vi "Main_15B.vi"() -> ()   [LabVIEW 2024]
uses:
  Utility/Universal Utility/TypeDefs_Utility/Cluster_Row-Column.ctl
  Utility/Universal Utility/TypeDefs_Utility/ENUM_4 Directions U-D-L-R.ctl
  Problem-06_Guard Gallivant/ENUM_Direction.ctl
  b5234449-2328-4583-8824-3fa0b55a92a1.vi
  51507f66-8fb0-4352-a9b4-7069ff2e9da3.vi
  afbcc12a-728a-4e4e-a13e-cfea6d256629.vi
  <vilib>/Utility/error.llb/Trim Whitespace.vi
  <vilib>/Utility/error.llb/Trim Whitespace One-Sided.vi
panel:
  out "Direction":T1
  out "Grid Start":string[][](array[string])
  out "Array 2":T1[](array[typedef])
  out "Position":T2
  out "Grid End":string[][](array[string])
  in  "Example 1":string="#######\n#...#.#\n#.....#\n#..OO@#\n#..O..#\n#.....#\n#######\n\n<vv<<^^<<^^"
  in  "Use Puzzle":bool
  out "Answer 1482350":u32
  in  "Puzzle":string="##################################################\n#.......#....O....O......O..O#.OOOO....#.OO......#\n#..O.O..#O..#O..#O.OO......O....O..O....#O.......#\n#...O......O...O...O.......#O#.O.#OO.O........O.O#\n#..O..#O..#.O....OO..OO.....#.OO.....#.O#OOOOO.O.#\n#........O#.....O..OO......#.O..O#...O.O..O......#\n##O..O.O...#O.#...#O...#O..##......#............O#\n#.OO#O.O..O...O#..OO...#..###O....OO.#.O.##....#.#\n#.O...........O.....O..O.OO.O.O...O..OO....OO....#\n#OO..........O...O........O..##O.OOO.O..O..O..#.O#\n#.#O.....O.OO....#O..O...O.....O...........OO..#O#\n##.....O.......O.O.O....O.O...#O.O..O##....OO#...#\n#.OO......O.......O..#...O......#.OOOO.OOO...#O..#\n#.........O.O....OO..##.....OO...#....O.OO..OO...#\n#O....O..O..#...OOO...OOO#..OO......OO..O....OO.O#\n#....O.........O....#.#.O..OO......O.O..#O.O#OO..#\n#...O.OOO.O.O..O.........O.OO....OO.O.....OO..OOO#\n#..O.........#...OO.O#.O....OOO......O..........O#\n#........O.O.O.O..OOOOO.#.O.OO#OO.....#...O.O.#O.#\n#OO...O.#O.OOO....O....O.#.O.OOO.O..O......OOOO.O#\n#...#OO.O..O...O.OOO.....O.O.OO.#..O#...O..OO....#\n#O.OOOO.O........#O.##......#....#...OO..O.O.OO..#\n#.OOO.O.O#OO...O.O...O.........O........O..O#OOO.#\n#.#..O........#......O......O.....O....O.#..O....#\n#...#.....O.O.OOO.OO.O.O@O.O.O.O..#O....#.#.OO..O#\n#O.......#O...#O....O.#.....OO.#O.O..O.O......O..#\n#......O...OO.OO..O#....OOO.#.#....O.O....OO....O#\n#...O.O.#..OO#.O.OO...O.#.#..#O..#...##..O.......#\n##O...O..OO.O..O.OOO..O.........O#O...#..#.O..O#O#\n#O.O....#OO..OOO.#O..#O..O.#...#.#..O....O.O....##\n#.O.OOO.O....O...#O.O...OOO..O.....O.O..O.O..O..O#\n#......O...O..OO.O........O..........O....#....OO#\n#.O..OO.O.OOO..OO...........O........O.O....OO.O##\n#.O.OO#....#.........#..O...OO...OO..OO..........#\n#...OO...OO..OO.O...O.....#...O.#.....OO.O.O.O#O.#\n#OO......#...OO......O..O.O...O...#.....O......OO#\n#O...O.....O...O.O.O....O##OO.O..#..O....O#OO...O#\n#.O.O#OO..##.#O...O#O..O.O#..O...OO...OOO.......##\n#...O.#.O.#......OO.......O.OO..#.OOOOO...OO..O.##\n#............O..O.....#O.##.O.O.#....O#.......O.O#\n#.O..##..O....#O.O..#....O...OOO#.#...#..O...O...#\n#.O.OOOO..#.........O.O#....O....OO.OO.....##OOO.#\n#..O#...OO..O...O#...#..OO.OO...#....O........O.O#\n#.O.O..O....O...O.O.OO#...OO..O.OO.O.O..O...O....#\n#.O#..OO...#.OO...........OO.....OO#O.#..O.O...#.#\n#..................O.......O...OO..O..O.O.O.O##..#\n#.##.#..OO.#..........O#...O.O.O...##..O......O.O#\n#OO.O........####.......O.......O......O...##....#\n#.O........O..O..#...O.OO...#....#.#.....OO...O.##\n##################################################\n\n<><v>^vv<^<v<>^>^^<^^>>^>><vv^>^>^<v<>>^^>>v^>^<v><v><v>>^<^<<^^>^>^<<v^<<^^v><<><v>v^>^^<v<<<>v<>^>^^^><v<><v^<><vv^v>^>^>><^<vv<^>^<^<<<<<^<^vv><v>^v^^><<>>v<v>vvv^<>v<>v><<<v^<^<^vv<^v<>v<<<<<>v<^<<<^<^v^<^>^>>vv>>^^<>^^<^v<^v<<vv<vvv^<^^<>v^^><^^^v^>^>^^<<<^<v<^<><v^<^v^<>>v><^^v^vv><vv>^v>>^vv>v><v<>>>^>>^v>v^^<vv^<v>vv<^<>^>>^v^v><^v^>>^>^<<<<<><v<v<vvv><><^^v^^^<>v<>vv>v^>>>^<>>^^^><v<^<>v<^>^<vvv^>^>vvv>>v<>v<>v<><><<^vv>^<^<<>^^<v<^^>v^v<v<>>^^><>^>>>^v^<>^^^<>><v><>v><>v>^<>vvv>>><><v<><>v^vv^>v^^>>v<^<^<v^>>>^^>>v<<<v^vvvv>^^v>^v<^>^vv^v^v<^^>v>^vv<<v^^^v^<v<^v^<v><v>^^v<^^><^^<^vvv<v<<><>v^<>><<<^vv<^^<<>^^<^<^>^<><v><^>v>><><v^vv<<>>^^>vvv^><<^v<<^>^<^<<><^<>^<>vv>><v>^^<v<v>v^v^^<<>^>>^^v>>v>^^>^<><^>v<vvv>^>v<><vv<><^v>>^<^^<<<<<>^vv<<<v>^<><^<v>v^<v<v<v^<v^<>^v<vv^vv>v^^>v^>^^<v^<<v>^^v>v><<<<<^vv><v>>v><^^^v<^^vvv^^>^^^>vv<>v^<>><><<><^>^^^v^<v>>>v<>vv>vvvv^>>v<<<^vv>>>^v^v><<^vvv^<<>v<><^v><>^v>>v>^^<<>v^vvv><^^<>>^<<<<>>^>>v^^<>>>>vv>v<v^>^<^v>v>>^^>v^^v<^vv><^<^^<vv\n<<^<><v<^vvv<<vv<vv<><v^v><>><<v^<>^>>^>>^^^<^^v<vvv^v>v<>^>><^v>^^vvv^<>>>v>>vvv><^^v>vvv<vv<><v>>vv^^<>^^<^>v^<v>vv^<><v<^<>^vv>^^><>^>^v^<vvv><>^>><^<^>v>v>><v<<vv^^^>^v^vvv>>vv^^<^^<>>v<<vvv^<^<^>>v>>v<<v^<^v><v^><^>v^<v<vvvvv>>>^^v><<^^>v><<<^^<<<^><^<<^v<>^<>v<<<v>v<v<<<^v^^^<v<^^^<^<vv<>>^<^<>v^>>v^v><^vvv>^>>v><<^<<v>v>v>^v<v^<v^^v>^>>^<v^v<>^v><<>>>>>^>^<v<v>>^^v<><><<v>vv><^<>><v>>>v^v<>^><v^v^><<v<^^<vvv<v>^>vvv<>^>>v>^v<^^^v>v>v<>>^<><^<^<<v^<^>vv^v^>v^^^^^v^v><>v<><<<v^vv^>v<v<><>>^^<^<v<>^><>v^^>^^><>v>v^^>v<>>^>^^<v<^^^<<^^>^^>vv<^<^><>^^^v^^^>>^>>v<<^v^^v^<^^^v<^^>>^>^<v<>>^^>><vvv>v<v<>^<vv<v^v>^<v>v>v<>v<v<<<><<<^>>>^>^v>vv>>v^vv^<vv>><<>>v^>^^>>^v>^^v^v^<^<v><><v>v><^^^>^><v>vv<><<^^^<v<^^vv<><v<v>vv^^><><^v^<^v>v<<v>>v<vvv<<^<<v<vvv>>vv<<^<vv><>>v><vv<<>v<vv^><><^v<^<><<>>v<>v^v^<v<><v>^>v>v^vv>v<<v^>>><<<v<^v<v^^v^^>v^v>vvv>v<^v<^<<^>v>><<<v<>>vv>v><vvvvv>vv>v^<^^^<v<v^v<<v^v<^^>>v<vvv<>v>>^<v>^<v^<>^^>>^>vv^<>v^v^<vv^<>>v^^^v^^^^>^v><v<>^>v<v><>>><><^v><^^v<>v^v^>\nvv^^>v^^v<v<vvv<v<<v^>vv<>>>^v^>v>^><>v^><><v^^<^>v><vv>>><v<>v<<<^v<<>^^<vvvv^^>v>v<^>v^^<<vv^v>v^><><><<vvv>v>vv^<<<vv^<v<^>v^<^>vv<>>>vv>^^^^>vv>v^^v<>^^^>v><>>v<>v>>v<^<<>^>><^v<<^<^>><>vv>^><>^^^^^^>^<^<v<<^<<v<v^v>^vvv^<>^v^>><<<^^>^^<v>v^v<^>>><^^<v^<vv><<vvv<<^>v^^>v>v<v^v>v<^v>>v^>^<<v><v>^>^<v<><^>><>>^><^<<^v><^<<>v>><>v<<v<><^v>><^<vv>>v^<><>>^^<<v>>>v^>^v>v>^<v<>><v>^<v<v^^^>^>^vv^<vv<<<>><>><^<v<<<v>>v>^>^>v<><><^v<>><>vvv>^><<^^^<vv<vv><>vv>v^>vv>v><><<^vv>^vvvv<<<<v<v^<>>v>v><v^><v<<v>>^v^^v>^v<<v^^>v>><v<<v<^v<v^^<<<v^^<<v^>^^^^^^<><^>v^><><v^<^^<>>v^<v^v^^^<v^>^^v>v<>^><v>^^><^>^>v>>^<>vv<v<^^v<^^>v^^<>^<^>>>^<^v<vvvv>^<v^>v<<^^^<v<>^v<<<>>^<<^vv>>vvv>v<<>><>^^><vv><<<^v>>><<<vv<v><<v>^v^vv<v>^>>v<<v>v>>><v>><^^v^v^v<<>^>v^>><v^>>v><<vvv^<^vv^v>>^^>v^v<<<>^>v^^v<<vv>v^>v<<^^<<>>v<<v<v^>>^><>^vv^><^>v<<v><<<v<^vvv^v^^v^>><v>vv<>^>v^<<v><><v<^v>v>vv^^v^^<<>>^<v><>v^>>>v<^<vvv<<v<>v>v<v>vvvv>^v>v>^^>v>^><v<^>v><<>><v^vvv<^^v>v^^^^>^<v<>>^>v^<^<>^^>>><v^v>>^><^v^vv>^<v>v<\nv<^^vv><>><<^v^<^v^>^^<^>vv<<^vvvvvv^<><<vv>^<^v>>>><^v<<^<>><>><>>>><<^>>v>>^>^^>^><^<<v^v>v^v>^<^v^<>vv^v>><>vv>><>^<<v><v^v>v>>^^^<<^v><v<v^^>>^vv^>^^>^^v^<<<^>^>^><>v<<<v^>^^^>v<>^<v^v<>>><<<v<>^>v<^^<>^^v<^v>>^>><v<v>>^><^v<^<><>v>v>>>^<<><^^^<<<vvv<^>>^><^><v^<v<v><^v^v<<<><v<vv><<^v<v<<v^^<^<^^^>v^^>v><>^v^><^>>>v>><^v^v>v^<<>v^v<<^<<vv^^<v^^v<>^>^>^<>v>^v<>v>>v>vv^vv>^><><v<^<><<<>>><<>^>^<v<>>>^^<>>^>v^><^vv><^<^>>v>vv<^<v<><^v<^>>><^v<^><v><v^v^<<^><^<><^^<^v^^v>vv^^<v<<>^>>^^v^^<vv<<^vv<vv^<>vv>^>^<v^><><<><<><^v>^^v^><<<v<^<vvv>^><<>>><<v><>vv^^>>^^><<v><^<v>vv^^<^<^^^>^<v<>^v^>v^^v^<>v^<v^v<v><^>v^^><<<>^^^<<v^v<<<<>>v<v^^v^vv^vv^v>v>>^>>^vv^v^<<^vv^<v^v^<>^<^<v>v^<<v<<>^^>><v^>v^^>v^>>>v><<>><v^^^<><><v<<v<<^v>v^>><v<>^vv>^><v<^v>^<>v<<><>>v^v^>^>v>><^<^^><v><^>vv>v<vv^><^^v>^^>v^v<>v<v^^^<<><v>^^vv>v<^>vv^^v^v>>^vv^<><^<^<<<v<>><>>^>^^^^><^v<<<>v^<^^vv><^v>v^vvv><>v>^<<^^^v^^<>>v<^^v<^^^>>^vv<v^^<vvv<^<<^>v^<>^^^<^v^^<v>^><^>^^^v^^>^<>>^v^>vv<v>^<vv^^><^v^^^>v<^v<<>v<^<v\n<^><vv^v^>>^<>>>v><^vv<v^<^vv<<>v^>v<v^^^^>vv^><<v>^^^v<v^<<v<v><^^v>^<v<<^>^^^>v>v<^^>v^v><<vvv^^^>vv^v>^<vvv<vv><<>>>v>v<vv<><<><^v>vv><<^^^vv<><^<<^>^><<>^<v>^>^v<<>>v^<^vvv<v^>>v<<^>^>v<<<^v<><><^^<>^<^<v><<vv<>>^<v^^><^^v<<><vv><^>^^>v^vv^^<>^vv>v^>v>^v>v>^>^>^>><>v<^v>><^<>^v<>vv<^v<^v^<>^<>^<^^v><v^<vv>v<^>>v>>v^v^<^vvv>><v<vvv><<^^<^v<^<vvvvvv<v^^^>^^vv^^v>>>>>^^>v^>^><^><>>^<>v^>v<<<^v><v<v^^vv^<^^v>^v^<vvvv^^<^<^<<<v^v^^<v<<v><^<v><vv<^^>v<vv<^<^v<^>^^^vv^<>^<v>^v^<><>><v>v^<<><^^^>>vv<v^^<v>>^<<>v<vv>^<<v<^<<vv^^<v<vvv>^vv<v^><vv<><v>>^^>v>^<>>^^<v<v<v^<vv>><<^><v<v^<<vv^^^<v><<^<v<<<v>^<vv^><<<^^v<^>vv<>>^>^v^<v>^^v>>v^>>v>vv><<v<<v>v^vv^>vvv^^v<>^>^v><vv>^><v>v^>^v^^><>v<^<v>^<<^vv>^v<<><vv>v^>vv<>>^>>>><<^v<v>^<><v<<<<>>^v>v><^v^^>^<<<v<v^^v^<>v><^>^>^^^v><<<^>v><^><<^vvv<vv^v>v^><<><^>^<<vv^>v><>v>v<>v<vv<>v<<^v>^>^v>^^v<>v>v<<v^v>>>vv>>v>>><^^^v^>>vvv^^vv><^v^<vv^><<^v<vvv<^^v<<vv<<v<><vvv<><<>v<v>^><<>><v<v<>^<v<>vv<<><<v^>^^^^^><<><^v^v<^>v<^^^><<<^<^v><^v<>^>>v^v^<^^\n>vvv^<<>vv>vv<^^vvv>vvvv^<^>v^<vv^^v>^v<<^<<v<<vv>^v^v<<><v<><<>>><><v><<>v<<>>v<<<^>><v<v<>>>>vv>>>>^v<>^><v>>^><v<>^v^v<>^v<^v>^v^^v^^v<><^v<<>^<>><v><^<^<<<><^v^vv<<<<>>>^vv<<><<v^^vv<>vv^>v<^v^>vv<>vv<<v^<>^<<<>^><v<vv><>^v>vv^><<^^<v<<v><>^>>v><>^>vv^^>>^^<^>^^<^vv^^<>><v<<^><<v^^^<v^v<<>>>>^v^<v^>>^><<v^<v^^>>v<<<v>>>^<v^^>v^v<>^>>>>>^^^>v>v>>vv<v^^>>^v>v^^vv<<vvv<<>^^v<<>>>^<><<<>v<>>^v^><<>^>v<>^^^>v>vv<vv>^<^^v<^^>v<^^^^<<<v>><<vv<v>v^>>><v^v>v^^^v<<<v^><>><^<^<^>><>^^v>v>v>>v<>>>v^^><^v<^>><v><v^<^<^>^^^>>>v^<>^>^v^v<vvv<^^^<>><<v<<>><^v>v^v<>>vvv<vv<<><v<>^<<^vv<^vv><>v<^v><^<>>>^<v<vvv<^vv<^vv><^v^><<<v^^<<^v^v>^>v^^^^v<>^^^<<><<vv<<^>vvvv^vv>^<vv<^^<^>^<^^^>v>v^<<>^>^<<v><>^v^^^><<><>v><<<><>v^>v>^<<<>v^>^<<^vv>>>^vvv<>>vv<vvv^<v<>>>v^vvv^v>^>>v<v^>><v^<^<^<^v<vv>v>^><><><^v>>v<^^^v>^vvv^^>>^<^<^^><<>^^<v<<^>^>^>v><>v<<v><<>><^v<>v>^<>^v^>v>^<>^>^>v^<v^><<>><<>v<^v>^<<<<<<v><<>><>><>><^v^^^vv<v^v<vv>v>vv<v^^^v^><v^^v<>v><<>v>>><<v><^<><>^v<v<><<<><>>^<v^<v<v<v^v<v<><v^<>vv\n<<<v^>v>>^>v>v<v<>^^><<^^><^^vvv>>>^>^><<^^<v<><v<<>^^^^vv<^<v^><<v>>><<<<<<<vv<<><v<<<>v<v<<^vv^<v>^^^^^^><^vvv<>v^>^^vv<vv><^>><v<>><>^<<vv^^<>^>^><v><v>v<^v<v<^^^^><^<^^><^v^^<vv^<><<^>^v<v^^v^^<>><<v<^^^<>vv<^^vv^><v><<v^v>>vv^><v<^^^v<<v<<<>vv>>><v<vv>^<^<v<v<>^>v><^>v>v<^<>v^^>>^^<>^<^<v>><<^<<^^^v<v<^<^<<v<v>>^<>><^v^v^<>vv>><v^^><v>><^<^>>^^<<v^<<<>v<^<v^v<v><<^v<vv<v<<>^v^v<<><v^><>><^v^vv^>>v^^v^^^<v><<<v>>^v^><^<v<<>>>^v>^^v<><vv<^^<>^^<<v<<v<<v^^^<^v^<<>vv><<<vv^^<^^vv<^v>^<v>^^^vv^<>v<<>^vv<<vv^^<>v<><^^<vv<<v^<<^<^vv>><^>><>><v^<<v><>^<<^vvv^>v^^>v>v^^^^^^^^v^^^v^<^^^v^^vv^>>v>v^^<v><><<^>v>><^>^v^><^^v>v^vv<v^>^>^<<^^^vvvv<<>><>v<>vv<vvv<<v^^v^^vv><<>^<^>^^^^^vv>^><^^^<<><>^^v^>^^>>v^^^<^<><>^<<>>v^<v<^v<>>>^<vv>^v^>^<<>^v<<v><^v^>><>^<><<v<>><v<>^>^vvv^^>v^>>v>>^>vvvvvv>>v>^vvvv>>^^^<<v>^^^<vvv<<v<v^v^^v<><<<v^v<><<vv<<<<vvv^^^<^>v^v^v^^>^v>^<>^v>>><^vv>vv<^^^vv<>^<><><>vv^v>v>v>>>^v^<^<>^<v<v<v><^<<>^^<^<>^v>>^v^>v^>v^>v<v^>^<>v^<^<^<vvv<v<vv^v<<>>^<^v<^^^<<<^>^^>^<<v>\n^v<v^<^^>>^v><v<><^<><><>v^<>^><>v<<vvv<><>v<><<^^vv>>^^^><^^<>^>><<^^>v><v><^>^>^>><>v^<><><^^^v<^<v^<>v>vv>v>^<><<><^^<^^v<><^<<v^<<^>^^>>>^>>^^^^<^v><><<<^^<^v>v^<^v^><v>^^^><^>^vvv>^v<>v<v><<<^v>^<v<<>^^^<^>^^^<^<v<<>>>>v^>^v^>v^v<v<<^<^^<v^^>v<><^<><^>v^v><<v<v>^vv<^vv><v<v<^><>^v^<<^>vv<^^v<^vv<>>v>>^<>^>>^>>>>^v^<>><v^>vv^^>^v^>^<<<v>^><<>>>><<>^v<<>>>>>^>^^^>>><^>>v^vv^^v><vv>^v^vv^vvv^>^>v>v^vv>^v^^<vvv>vv>><<<<^<<<><>v^v^^^<>^v^<>><<^^^<>vv<<<v>v<<<^>><>^<><v<v>v<v<vv^vv<v^vv^^<<<<vv<>vv^vv<v<<v<v><><>^^><^>^<><^v^>>^<^>>>vv^><<><<^>><v<<v^v<>^v^^v^<><v>^v^^vvv<<v^v<<^^^^^<vvv<><^<>^v<<>><v^v^>>>v^^<^>v<><vv><<<<^<v<v<<<^>v<<<v^v<<^v>^^><<<v>vv<<>v<>v^v<^<>^>>><^v><>^^v><<>vv^v<^v><vvv<<vv<><^>>>v<v><<^^<v>^vv^^>^v<<^<>v^v<v><<>^vv><<<vv^v<>^<v^v<^v>^<<<>^>^vv^><>v^<>v<>>>^vv<vv^<^v^<v><>>v><vv<v>><^v^^^^>>v^>^>v^^<<^^v>vvvvv<>^vv^<^<>^<>v>>vv>v>v<>^><>v^^^vv^>v^<>^vvv<>>>v<<vv<<v>>v>><<^vvv^>v^<<v<v<<>^<><^v<<^>>>v^<^>v<<<<v>^^^^^v><>v>vv<>>^<v^^^v<>v<<>v^<>>v><^^^v^^^>^^>v>\n<>^^<<vvvvv^>vv>>>^<>^v^vv<v^<^v>^^><^>><<^^vv>v<v><v^<^<^>><><<<>v^v>vv<v^v^v>><><v>>^<v^<><v<^^^v<v<<v<<^>^v<^^>^^^vv^><>>^<<<<v<^^<v^<<^^<v>>v^^vvvv^vv>v>>vv<^^>v^vv<>v<v<v<^<v>v^>v^>>^<v><<<<<^^<>>^v^<<v^><v><>vv<v>^^<^<><v<^v<^^vv^<><v>^<<^<>^^^^^>^vv>v>^>>vv>v<>v^^<><^^>^>><>^^v>v><v<^<<<^v<>^>^v^^v>v>>^>^vv><^>^>^<><^^v><v<^>v>vv^v>^v^>^>^v<v>>v>>v^<<v^>v^>v^>>v<^<<<><>^vv<>>v<^^^>v><<<><<<vvv<v<>v<^vv^v<v><^^vvv>^^vv^<>>v>^vv^^<^<>><<>v^v^^^^^<v>v^^<<^^<^v>>>^>^^^^v>^^v><^v^>^v>^^^<>^<<^v^v>v><^^v>^vvv<<>>^v^^>^>^v<v^>>>^v><v<>vv^v>v>v^v<^v>vv>>^>v^<^^^^>^<^>v^^>>^<>^^><v>vv<^>^^<^><<>>^>^v>>v>^<^v<<vvvv^vv<>>v<><^v^v>^v^^v^v<v><<^^v><^>^>^v<vv^^^^<^^v^v<v>^><<<v><<<>^v^>v>vv<^<><^^<>^<>>vv<v<<>^><^^^^v>v<>>v<<>vv^>^vv><<vvv><>v><^v^><vvv>vv<v^<>>^v^^<<<<>>><v<>>^^><^><v<^^<<<<^^^>vv^>^v<<v<vvvv<>^^v>^>v^^><<^<^v><v>^^^>v^<>>^>vv>><^^><^^^>^>><^<>>>>vv><><^<>>v<>v>^v^>^>^><v^^>v>>>^v^vv>v>><>v^^^>><v><>v<>v^^^vv<<vv<vv><><<^<<<>vv<vv>v>^^<v>>v^>>v><<v>^^<><>^>v^<>^vvv>^<^v<<vv<\nv><^^>v>v>^<^<^<<v^<<v><^^<<<^^>><<<^>^^vv<^>vvv<>^^^<<>^vv^v>^^v>^v^^v^<>^vvvv^>vvv>^^<<v>v>^>vvv>><<<v>>v^><>>^<<v^<^^v>><<^^^^><v^<<^^>^^v>^vv^>vvv>v^v^vv^>>^<^<>>v<v^v><<^^^><^^vv^v>v>^>v<v>^><>^<>^>^>vvv>>^<^>^vv>^^<>^^>^><^>^<v<>>^vvv<vv^v>>><<<v^>^v^><^v^<v>vv<<<><<<vv^^vv>>v<v<>v<><^^vv<>>>^v^^<^<<>^<<^<vv^<v>>>v^<>^>>vv>>>^^v^v<vv<^v>v<<^v<^<v^v>v<v>^^><>v^v><<<<v<>>>v^vv<^>>^><v>^v>^<vv<<^>^>v^^<^^^^vv>><v^^v^>^>><^v<^v<>v^>v<<^<v<vv<<^<>vv<>^<v<>^^vv<^^^^<^>^^v>v>v>v<vv>v>v>vv^^<^^<vvvv>v^<^>vv>>>^^^>>>><^^<^<v>v^^v>>>>>v>^>>vv<v^>vv<<<><>v>vv>^><<>>v^<vv<v^v>^v^>>^v^<>^v<^v^<v<^v><^^>v<v<>>><>><^>>^v<>>><><<v>^>^<v><^<^<<v^>v>vv>>vvvv<^>^><>v^<>^><<v^^^^^v>^>v<v^v<>>>^^vv>v>><^^<>><<v>vv<<<>><^v><v>^^<vvv^^^^^<^v>^<<v>>^^vv><<<v<>v^<<><v<>><^<>v<<^v><vv>>^^^v>v><^^<v^><^<v>vv<v^^^^^>><>^^<<>^>>v^^>v^<><>^v<^v>>v^vv<>v<<^<v^v>>^>><v<^^vv<^^<^<v<><^vvvv^>v^<<<><<v>^^^><^><v>^<<^^vv^vv>v>v<^>>>>^v<^v>^v<<^>>>^<<^<v^^v<^<v^<v>^^^vv>^<>^<^<^><vv>>>^<>^^<<<<<v^^>>>vv<^^>>>v^<vv<^\n>>^>^^>vvv<<^^vv^<^>v>^<^<^<^>v^<v>>v>>v>^^>^<<>>vv>>^>>>>>v^<v>><v<>^<vv<>>><v<^^^v<v^<v^>^>>>v>^v^v<^v<>^^v^^^>>>^>v<^>^<<><v<<<<v>v>^<^^^<<>^<v^>>^<<<^>>^>^^>^v^^><vv^<v<v^v^<^>^<v^vv>^><^^^><^v<<>v<^<^<v>^^>v>^v><>^<>v^v^<^<v><>vv<>vvvv<<<^v>v>v^^<<vv<<<<v>>v^^^v>>v><^^^><v<<^v^v>^<<>>><^^v>>^v>><><><<vvv<^^>^vv<^^v<>^vvv><<^^<v>>>^>vvvv^^vv<^v<v<><<vv><><>>>><><v>v^><^vvv>v<<>^^^v>><vv<v<^<v^^<<>><<^<><vv<>^><>>><^v>^<>>vv>><>^>^<>v>v<v>v^^>^^^>^><>><>v<<v<<<<v<<<^v<<<<<^>^v>^v<<<>v>><<><v<<^<>v^v^^v^^<^>>^^^^v^<<<v<>^^<^>>>>^^vvv<><^v<<^^>v>v>^v><v^<^>^^^^><<>^>^v<^v^><<<>^<^v<<v>^<^^^>^^^^^<^^<v<>vv>^<^<<vv<^^>v^vvv<^<vv<^><^^>^^v<^v<><><>>v><v^<><^vvv^v^vv^^<^<^<<><^<^<>>^<<<^^>v><<v^>^v<>>>>^v<^>^^^^v>>^v<^>>v><^^^<<^<<v^>vv>v<^^vvv^v>><<>^><<^v<v><v<><vvvv^>v>>v<^>^>>^<^v^>^v^v<<^<^>^vvv^>>v>^>v^vv>>><<<vvv<v>^><^>vvv<^v<v<<v<v^v^>>^vv^><v>^v>v>v^v<^<v>^vv>v<v>v>>>^^<vvv>>><<>^<>>^<v>>^^^<^^v^v><>>>v^^^vv>>^<^v^>>^v>>^<>vv^vv>^^><v>v><>^><<>^<>^^^<><^><v<<<<>>>v<<<v^^^v^^v>^<\n>^^<<>v^><v>>^v^^<v<^<>^>^v<><>^><<>^^>>^^>><>>vv<^v<^<>^^v^v^v^^<>v<<><^vv^>vvv<vvv<v>v^v^<<vv<v><^^>>v<v>v>^vv>^^^v<v<>><v^>>v<^<v>v^v>vv><>v<>>><v^^<v<<v>><^>>><v>>v^>^v>v^^v<>vv^><^v^>^^^vv<v^>v<v>^^v^>>^v<>>><v<^>>v^<<^>>>^<^>>vvv><>^<v<v<^>^^<^<>>^^v><>>><>vvv>^<<v>><>>^>><^<v><^><>^^^<^v><^^<<<<^<<^v<><vv^><^^^>^<^<<><vv^>v^<^>><>>^><^<>^>v><>>v>>>vv>^vv^>^^><v^^v^<<>v^^^vv>v>v^>>v^<<<^vvv><><><vv<><>^v>v^<>>>>^>><v<^^^vv^^<>v>v<^v<<v^<^vvv<<><<^v>vvv^^v^^><^<^^<<v^^<<^<^<<<>v<v<><>v^>vvv^<^^^v^v^v^<><v>vv>>v>vvvv^>>^v<^>>^v^^^^><^<v<^^<><^^<<<><>vv<<>^^vvv><vv^v<v<>vv<<>v<v<v^v>v>><^v<<^>^>>^v^<^vv><^>v<^v><v>^^v>><^>^>^^vv^>^v^^^v<v<<<<<v^>v><>><^v^vv>>^>><^><>v<<>v<<<v>v^^<<^>v<^><^^^><<^<vv<vv<<>^>vv>v><^><<^<>>v><<<^v^^<<<vv<>^><<>v^v>vv<<v^v>>v<<v^^vvv^<>><^v^<v<^^^^>>>>vvv>v^>v>^v>v><^^^<v^^>>>v<v>^>^^>v>vv<>>v^^v^>vv><<>v^>^^v<<>vv^^^><<^<>v<vvvvv^^^>^vv><<v<^>v><><><<v^>^>^v<vvv>v><v>><<>><<^<^<v>>v<v<^<><<v^>>>^>><^^^>^^<><v>^^<^<<<v<^<v>v>>v<v>>^^v^>v>>^v>^^>><<>v^><>\n^<v^>^>v<<^^<<<vvvv<^v<v^^^><vvvv^^<>^>v>vv<v>^<<><><^^^v^<^>^>>^^<^>v>vv><^^>vv<>^v<v>^v<^v>^>><<>^<v><v^>v<>^^vv>>^vv>^v^^v^^^>>>^<<>v><><<^<><^^^vv<v>v^>>^><>^^^<<^^v<^vv<<>>>^v<>v>v^<v<>^v>vvvv><<<^v>^>v<vvv<>>>^<>^<v^>^<<^v>^><^<^<vvv>^^>v<v<v<>^vv>^>>>^v^<>^<vv<>v>v^><v<^^<><v<>><vvvv^<<^<^<^v<^<^>^v<><^<^<>^<v<v^<^><v^>^v^vv>>^<>v^<>^<v>v>>v>><>v<>>^<v>>v<vv<v<v><>^<>^^>^vv^v^<v>>^^^v^>vv^^>^^^<<^vv>^<v>vv<^v>^v<^><>>^v<v<>v<v>^v^<v>v>>v^v^>>^^^>^v<^v>^^v>><^v^<>^<v<<v^^v^^><^^v<><<>^v>^>vv>^<>><v>><<<>v>^v^>v>^><<>v<v^^v><^v>^^<^>^^v<vv><vv><><^<>^><^<>>^^<<>^v^^>^>^v<^^><v><^^^<<^><<v^<^v<<v>vvvv>^^v<v^v<<>v<<>^v>>vv>>v><>^^<v>v>v>>^^>^<vv<^v>^>v<<^>^vv<<<v<vv<^>v>v>^^<v<vv>^><^>^v><v<<^v^v^>^<<^^v<<v>^v^>>><^>>^<^v<^v^>^v<>v<^v^<^^><><<^^vvv<^><^^<v>v><v>>v<^>vv^v><^^^v^<>>vvv^v<^<<>v><><v^>^><<>^<v<<v^<v^^<^<><^vvv>^^>v^vv^>vv<v<<>^><<<<v>>v^<>>v^>^><vv^v^<^><^vv<^>>vvv><v^>v^<><^>^^v<^>^>^^<<^<<>><^v^>>><^v<v^^^^v<><>>^v^^v<<v<^<vv>>>v^>^v<<<>^v<<><v>>v<<<vvv>v>><^>><vvvv^^\n>^^v<v^<v^<<v<v>^<<<^^><<>v^<^^<>v>^>vv>v>v^>^v^>v<>v<vvv^v>>v>vv<v>vv^>^><^^vvv<v<<><>^<<>>^^^v>>vv^vvv^<<v^v<v<^<<<<<<v>>>>^^^>>>>>>^v^><<v^<v<>^<v<v>>>^><<<v><^^<>>v^<^>^<>v^<^>^>^v^><^<^vvv>v<^v<>vv^^^>v<v>vvv<^<v<v^<<<>^<v<<^^<>^^>v^<vvv^<v^v>><<v>>^v>v>vv<><>>v<^v^><<v<v<^v<v<<><^<^>^<v<>>vv>v>^>v>^<v^v<^<^<<>vv<v^v^^v<>^^><>^<>vvv>>^^^>v>vvv<<><^v>>>^v^<v<><^^^vv>^^v>v>>v><v<^^^>v<<>^><^v<v<v^vv<><>v><<<<^v^>>^v>vv<>v^<vv^v^<^^>vv><^v^^<v<><v^<><^<<>v<<><<>>>^><<<v>^<^<v>v^^<<>>>><<<<<^>^v^v^>>><><>>>>>vv<<>^<v>v^vv><<^^<><^^<^^><<vv^<^v^^vv>>>>v>vv><>v>vv>v>vvv^<v<<^v<>v<<v><<v><><^^^^^>^^>><^v<^^<vv<<<<^v><<^v^<>>^^v<v^vv<><<vv<v<^<v<<><v^v>v><>><>v<^<v<>>>^><>>^^v>>>v>v<<><^<<vv^^><v<v>>vv><<>><<^>v^^v^>>>^v^<>vv<vv<vv<^^><<vvv^>^><^^v>^><>^<<<v^>^<v<<vv><v<^v<<v<>>><<><><<<vv>>v>>><>^v<<<^<^<^^^<<vvv^^>v<v^v<<^<><<v<^>><v<<v<^^v^v<>><<<>>^^^<v>>^<v<>^^>v^^^^<>vvv^<^<<<^^^>^<>vv^<>^^^^^<v^v>><<^<^^<^^vvv>v><<>>v^<<<>^^^><v>^>>v>^^><v<>^v>v<^^>v<^<>^^^<>^<>>v>^v><>v^<^>^>vv<v^\n><<^v<>v^v>v>^^>v^v<<^<<v^^>v<v<^>>^<v<^<>><vv>><<<^^v><v<><^>^<<>^>v^v>>>v<v>>v>^v>>v>v^<^<>^vv^><v<^v<v^<^v^<>v^v^v^>>^><><<v>^^<><^<v^>>^<>^<v<<<>>>><<>>v^<^<^<v>^><^v^v^<<^>>^^<v>^^<>v^v><>><<v<v<>^>><>>vvv<v>^<<v>^^<>^v<<^<<^^vv<^v<^>^<>><^v>>vv>v<<>><<>>^><vv^><>v<v^v^^v^>>^v^v>^^<^^<^^^<<vvv><>^^^<^<<<<vv<><v><^vv<>vv>^^>>^<^^v^>^vvv^^<v>^><>>^<<>>>><><v<^<>^>v>^<>v^v<<v>>^^v<^><^<^v><<>>>><><v^<><>>^<vv>>><vv>v<vvv>v^<^vvvvv^v>><<<v^>^>v<<<>^v^^vv<>^vv>^<v><^><><^>vvvvvv>v<^<>>v<><v^><^<>vv>>^^v>>vv<v^>v^v>^^><^^>><<<>>><v>>^v>v><v<^<>>^<^vv><^v<<v<^<^<vv><vv<>^^^>^>>>v>^>v<<><^^<<>>>^>><<v<v<<<^^>v><^>v^<<v^<>><<^<^<>>v^vvv<^^v><^<^v<>^v>v^><>vv<v<v<^v>^^>vv^^>^<v><^<^<><v<v><>>>v^>><<<^<^>vv<^^^>><<<v>^>v<>v^^>vvvv^<<<<>v<><v^>>^>>v^^^<v><vv>v<>>vv<^<^><v<^^<v>v<<v><^>vv>^v^>v>v<^<<><>>^v<<>v>^v^>^<v><<>v>^^<><><v><>>v<<v^<v<^><>^vv<><>v^<vv^^^>v<<vv>>>>>v^<>>^><>>v<<>v<vv^v><>vv<<vv^v<>>^^<v<^v<v>vv>^>>v>vv^v>v<>><>>v^v>>^>v<v^>>>^<v<^^>>v<<<vv<<>v><<><^v<>>vvvvv^v><<>^v<v>^\nv>^>v<^v>v><^>vvvv<<v<>^^<<>vvvvvv<v<>^>>><v><v^<<^>^v<>v^>^<<v<><vv>^v^>>^<<v<v^>^>v<><v>^>^^v<^>v<>^><v^>v<v>v^^>^^<>^<<^<<<v>>v^<^>^>><v>>^>>v^<^vv^^^vv>v>v<v>v^>v>^><<^<><<<<>v<vvvvvv<><v>^<>^>>vv<<^vv>^>^^>^v>vvv^vv>>v<^^>^^>v^<<vv^>>vvv^vv>vv><>v^v<^><<>^^vv<<^vv><>^<>>^^^vv^v^>^>^<<vv>><^>>v^vv>^><v<<vv^v>>v<^<>v<v><v<><^^vv^^<^<v^v>>^<vv^<<v^<v^^^><<^>^<<^^^>>vv>^>><><^v^>vv<>^<vv>>v>^<<>><<v>^>>vv<>^>>>v<vv<v^>>>>^v^v^>v^<^v<<>v<<<v<^<>v><<^v^<<v^<vv<^v<><^<^>v^<v>^vv>>v<v><<<^v<v<v^^>>^>v^v^>><<>>vv>>>>v^v<<v^v>^>v<vv<v<<>v><<^<<>vv>^<^>v<vv^^>^^>^<^v<>^<^<v<v^^v<^>>^<><^<<>^>^v^v><<>vv^v<v><>^^v>>^v><<v^^^>^v<><^<^^^^<>><<^^<<<^<^<^v<>^<^<v>vv>><<vv^>vv<>>><^^><^vv>>^v^<<>>>v^^^<>>^^>>vv^<vv^>v>>v<>v><><v>vv>v<<v^<><<<v^v><v^^v<<vvv>^^<^v<>^><v>>>^^v^<^<>^^v<^<>>>><v^>^^^>^v>><v>>v>^>^v>><>v<v<v<>v<^^><<><>^v<<<><>vv><>v><<<>>>>v><<^<^^>v<v^v<<v<^>><vv>^>v<v^v<<^v^^>v^<v^vv^vv><^<v<^v<^<>v<v^>v>^>^>v><^v^<><<v>>^v^><><<>^>^^>^<v^>v>^^vv>>v<v>^<v<v^v^>^>v^v<vv<v^^vv<<v<<^>v>^\n^<<>>>v^^vv<>^<>v>^v>>^vvv<><v^^^<<^^v<^v<^><<<><v>^<v^<^^<^v>^>vv^v^vv^>>vvv<vvv<^><>><><^<v<^^><^^v^v^><vv><<^vv<^v<v<^v<^v<<v>^^<<><>v<>>>^v^v<>>v><<<<>><vvv<^<<>>>^v^<<<^v^>>vv^v<^<<>^^v>>^^^^<^>v<^v^<><v^<<<^v^v^v>^>^>vv><<^vv>><>vv><v<>^v>^>>vv<^^<>v^^<^v^<^v^^>v>>^<v<<>>>v>><v>^^v^>^<>><<>>v>v^>>><>vvv><>>>v>^<<^v<^v<^<>^v<^>>^<^^><^^v<^<^<>vv<<v<^^v^<<<>v<><>vv^v>^>v^<v>^^>v<<v^>>>>v<^<<v<>vv<v<^^>>v<^v^^^>^<><>^v<<^><<v>^<v^v^<^>^>vv<v^^^^v^^^v^<>><^>>v<^v>v<>>>^<^<^<v^>>^<<<v<<v^^<>^<v>>v>^<^^v<v>^>^vv>v^>v>>vv<<><v>^v>^v<<<<>^<<<<>v<vvv>>>>><<vv><>v<v^<><^v<>v^^<v^>^^<<><^><<^v<<^>^<v^<^v<^vvv<^^<v<>v^v<><<<v<>>><v<<v^><<^^>^<>>>v^<>>v>><>v><v^><^<>>v^<>v^<^>v^<^<<>v<<<vv>^>>v^<v^>^>v^^<<^>>^<^^>><v>><v<<v<<>^^^vv>vv<<>^<v^><v<>^v>^^^^>v>^^<<^<^<^<<v><vv^^^v^<>v>>vv^><<>^^^<^>>>vv<>>v>^<>^^^v<^vvvvvv^<^^>><^<^v^vv<<v<<<>^vv><>>^v<v^^><<v><v^>^v^v<^v>>v^v><^>vvv<<^^<v>^^<<v^v>><<<>v<^>>^v<v^<^vv^v>v>v<v<vv^^<^<>>vv<v<v^<>v>^>v><^^^^<>^>>v<>>^<v><^vvvv>vvv^>^v^<<v>^>>^<<^>vv<>\nvvvv^v^^^<<^>^^vv<<^>v>^v>^>^>^^^^^^>v>>vv^>>^^>^vv<vv^<v<<<^<^<<<<^<<v^^^v^<<><<>^>^>v^<vv<vv>^>>^^v<v<v>^^v^^^^v^<<>^<>v<>>^><><v>^<vv><v^<vv<v^>>^v^^vv^>^v><<^><^^vvv>^^><>>^v>^^>v><>>^<>><^<^>vvv<>v^<><><^v>><^>^>^^^v>><>^>><>^<vv<v>^<v><>^>^vv<vv^^^<^<v^^v>>^>><v^^<>vv>v^vv<vv<v<<<^v>^<v>v^<<^<>vvv^v<<v<<vv>>vv<v<v<>v^>>><><v><^v<<^><vv<^^>^vv>>v<>vv>v^vv>^<^v<<><<^>^>vv<v^<v<<><>^>^><v^^<<>^^><>v<><^^^><v><vv<^^vv><v<^<v<^vv^<<^>vv>^>>>v^v>v^>^>v^vv>>><v<v<<v^>>v^^^<>^>^>v>>^^^>>>><><^<>>^vvvv<vvv^^vvv^<vv>>>>^v^>vvv<vv>^><^><v><<v<^v><v^<v<<>>><<v<v<<^>^v^<v^^<>^v^<^^>><v^>^vv>^v<<v>>v>v<v^vv><<><<^><^<<>^<>>>^vv^^^>v<^^^v>^v<>v^^><vv<<^^>^^^v>v>v><<^^<>><><<<^><>v<^<<>><v<<vvv<<vvv^>v^vv<vv<>^^^<^<^><<vv>v^>>v<<v<v>>v<<v^<><v^^>^^<>^v<><vv^<^v<<<>^<<^^v>v<^vvvvv>v^<^><v<><<<^<v<<<v<vv<^^>^<v<v^>^>v^^v>>^vv^>v<<<v><>^v><v>v<>v>^v^v^<^>^>^^v>><v^v<v>><<>^^^^^<vv^v^^<^>>>v<<vv^><v^v^^>><>^>v^>v>^>v^>vv><v<^<^>^>^v^>v<>><<<>^v>>vv^v<<^v>>><<><<<>^<vvvv<v<^<<>vv<vv<v<><vv><<^^vv>^><\n<^^^<v><^<vv^^v^><><^v<^>v^<v<>^v^v>^^v>>v^^>^v<<<vv<^v^><vvv><^vvv>>><>><^>><>>v<>v<<<^^<>^^^^>>^<^v^^<v<><<<vv>v^^^>>^<><^<>>v>v^>^^>>^v^>^^^^>v<^><>^<>>v<^v^<<>v^v^<>^<<<>v>^>>v^^v>v^v>^>v^^>>>v<^^v^^>>v^>><^^<^<<vv>>v^<vv<<v<^^^v<<v<v<v<>^v><^>v^<^vv<>>^v<v>^>v>^>^>><vv<<><<vv^v>>^^v><^<^^<<^vv><vv><<^v<^^^^>>^><v<^v>>v>>^>^<><^vvv^^<v^^><^><^^v^<v<<^v<><^><><<^v<v<^<v>^>v<>vv>^^^vv^^^^^<>v<<>vv<>^vv<^<^>^^>^^<^v<<<>^<v^<v<>vv^<v>^v><^>^v^<<<^<>v<<^<vv^v<^v<v>>v^^v^^v^v><<v<vvv<^<<^vvv^^v>v<<v^>vv><<^<^<^>^>^<>><>v<><>><^^><<<v<>><v>^<<<<^<<^^^^v>><^^v<v><v^v<^v^v>^>>>>v<>v<v^v<vv>^^<v^^^<v^v^<<^>v^><>>>v<>^v>v^^>><>v>^v^<^^v^v^^^v>^><<^v^vv<>>>^<<<>^^<>^^^vv^<v^>v<<<v>v<>>><v^><<^>v^^^v>^<v<^<>^^>vv^>>><><<^<v^^vv^>v><vv^^v<^^><<v>v^>>v<v^^^<vvv^^<<<^><<^>><>^^v<^^v<^^>^<<>^vv^v^^<><>v>v^^^<^^<v>><>v^^vv>>^vv^^>><>v^vv>vvvv^^vv^><v^^^>vv>^vv<v^^^^^v>^^><v^<^vv<>>>v<>>>^^>><<>v<^vv<<><v><>v><v^<<<<><>^^vv^^<^v<^>>>>vv<<^<>v<^<><^v^<<v<<>^<<<>^>><^v<vv>v>><^^>>^>^<>^^>>v<>^<<^v<><v^\n^<>vv<vv^^>^<^<vv><>>^<^^>^>^<^^v^>><>v^>v>v>vv><^>^>^>><<>^><vv>vvvvvv<<v>^^<<<><<^v<<^^^<>v<<<<vv^^v<><>^v^^v^>^^><vv><^vvv^^<^v^><>v>v<>v<<v^>>^v^>^^^^>>^v<vv>>><>^<^vv^^<v^vv^^^>^>^v^>>^^>>v><>><v^<>>vv^>^>v>v^<>v<<^<<^>v<<v<>v>vv^>^>v^<v<>^<>^v<>><vv<>><<>vv^^>^>^^v^^>v>^<<^<><v>>^<>v><>^>>v^><^^v<vv^v<v^>v^^<v^>v><>v^^><<><<><>^^<^<>vvv>v>v<>v>^<<>>^v<^><<<vv^>^<<<>v<^v>><^^>>>^<^<>v^^^>>>>v^>^<><^<<^><^^^<>^^>^^^v><^^<^v<>><<>^v<><^<<^^>><<><<^>^<^^>^>^<<>>vv<<<>v<vv>^<>v^>><>v>^^^>^><<^^^>>^^v^^<<><^^vv<>v^<<v>v>^vv>>vv<v<v<v<>v^^<>><^<<v<><>^v>^>v>^^vv<>^v^^>>^<>^<<^><^^^v>^v><v^^<>v^^<^v<<<><><<vv<>^>vv>>^>^<>^>v<<v<<><>><^vvv>>><v^^<^vvvv^v<^><><<>v><><<>v><^^^v><^<^vv>>><^^<^v><^<^^<v><^^<v^vvv<vv>v<<>^^^v><<><<vv<^<<^v<v<v><>v^>^<<<<v^v>>>vv>v^^^<>>>^<v>v<v>^^>><v<>^vv><><<<>v><^><v<v<<<vv><<vv^<<>^v^v<<^<<>>^>^^vv^>>>v>^><^vv><v<vv>^>><<^>>>^>>^>^>>v^^v>^<v><v^<<<^v<^<<^<>v^<<^<<v<><><v>^^v^^v<<^>v^v^>v>v>v>><>><<v<v<<><^>v^<<<^>^^<<<>^v>><v>v<vv<><^><<^<v>^v<<v<^>^v^^>vv"
  in  "Example 2":string="##########\n#..O..O.O#\n#......O.#\n#.OO..O.O#\n#..O@..O.#\n#O#..O...#\n#O..O..O.#\n#.OO.O.OO#\n#....O...#\n##########\n\n<vv>^<v^>v>^vv^v>v<>v^v<v<^vv<<<^><<><>>v<vvv<>^v^>^<<<><<v<<<v^vv^v>^\nvvv<<^>^v^^><<>>><>^<<><^vv^^<>vvv<>><^^v>^>vv<>v<<<<v<^v>^<^^>>>^<v<v\n><>vv>v^v^<>><>>>><^^>vv>v<^^^>>v^v^<^^>v^^>v^<^v>v<>>v^v^<v>v^^<^^vv<\n<<v<^>>^^^^>>>v^<>vvv^><v<<<>^^^vv^<vvv>^>v<^^^^v<>^>vvvv><>>v^<<^^^^^\n^><^><>>><>^^<<^^v>>><^<v>^<vv>>v>>>^v><>^v><<<<v>>v<v<v>vvv>^<><<>^><\n^>><>^v<><^vvv<^^<><v<<<<<><^v<<<><<<^^<v<^^^><^>>^<v^><<<^>>^v<v^v<v^\n>^>>^v>vv>^<<^v<>><<><<v<<v><>v<^vv<<<>^^v^>^^>>><<^v>>v^v><^^>>^<>vv^\n<><^^>^^^<><vvvvv^v<v<<>^v<v>v<<^><<><<><<<^^<<<^<<>><<><^^^>^^<>^>v<>\n^^>vv<^v^v<vv>^<><v<^v>^^^>>>^^vvv^>vvv<>>>^<^>>>>>^<<^v>^vvv<>^<><<v>\nv^^>>><<^^<>>^v^<v^vv<>v^<<>^<^v^v><^<<<><<^<v><v<>vv>>v><v^<vv<>v^<<^"
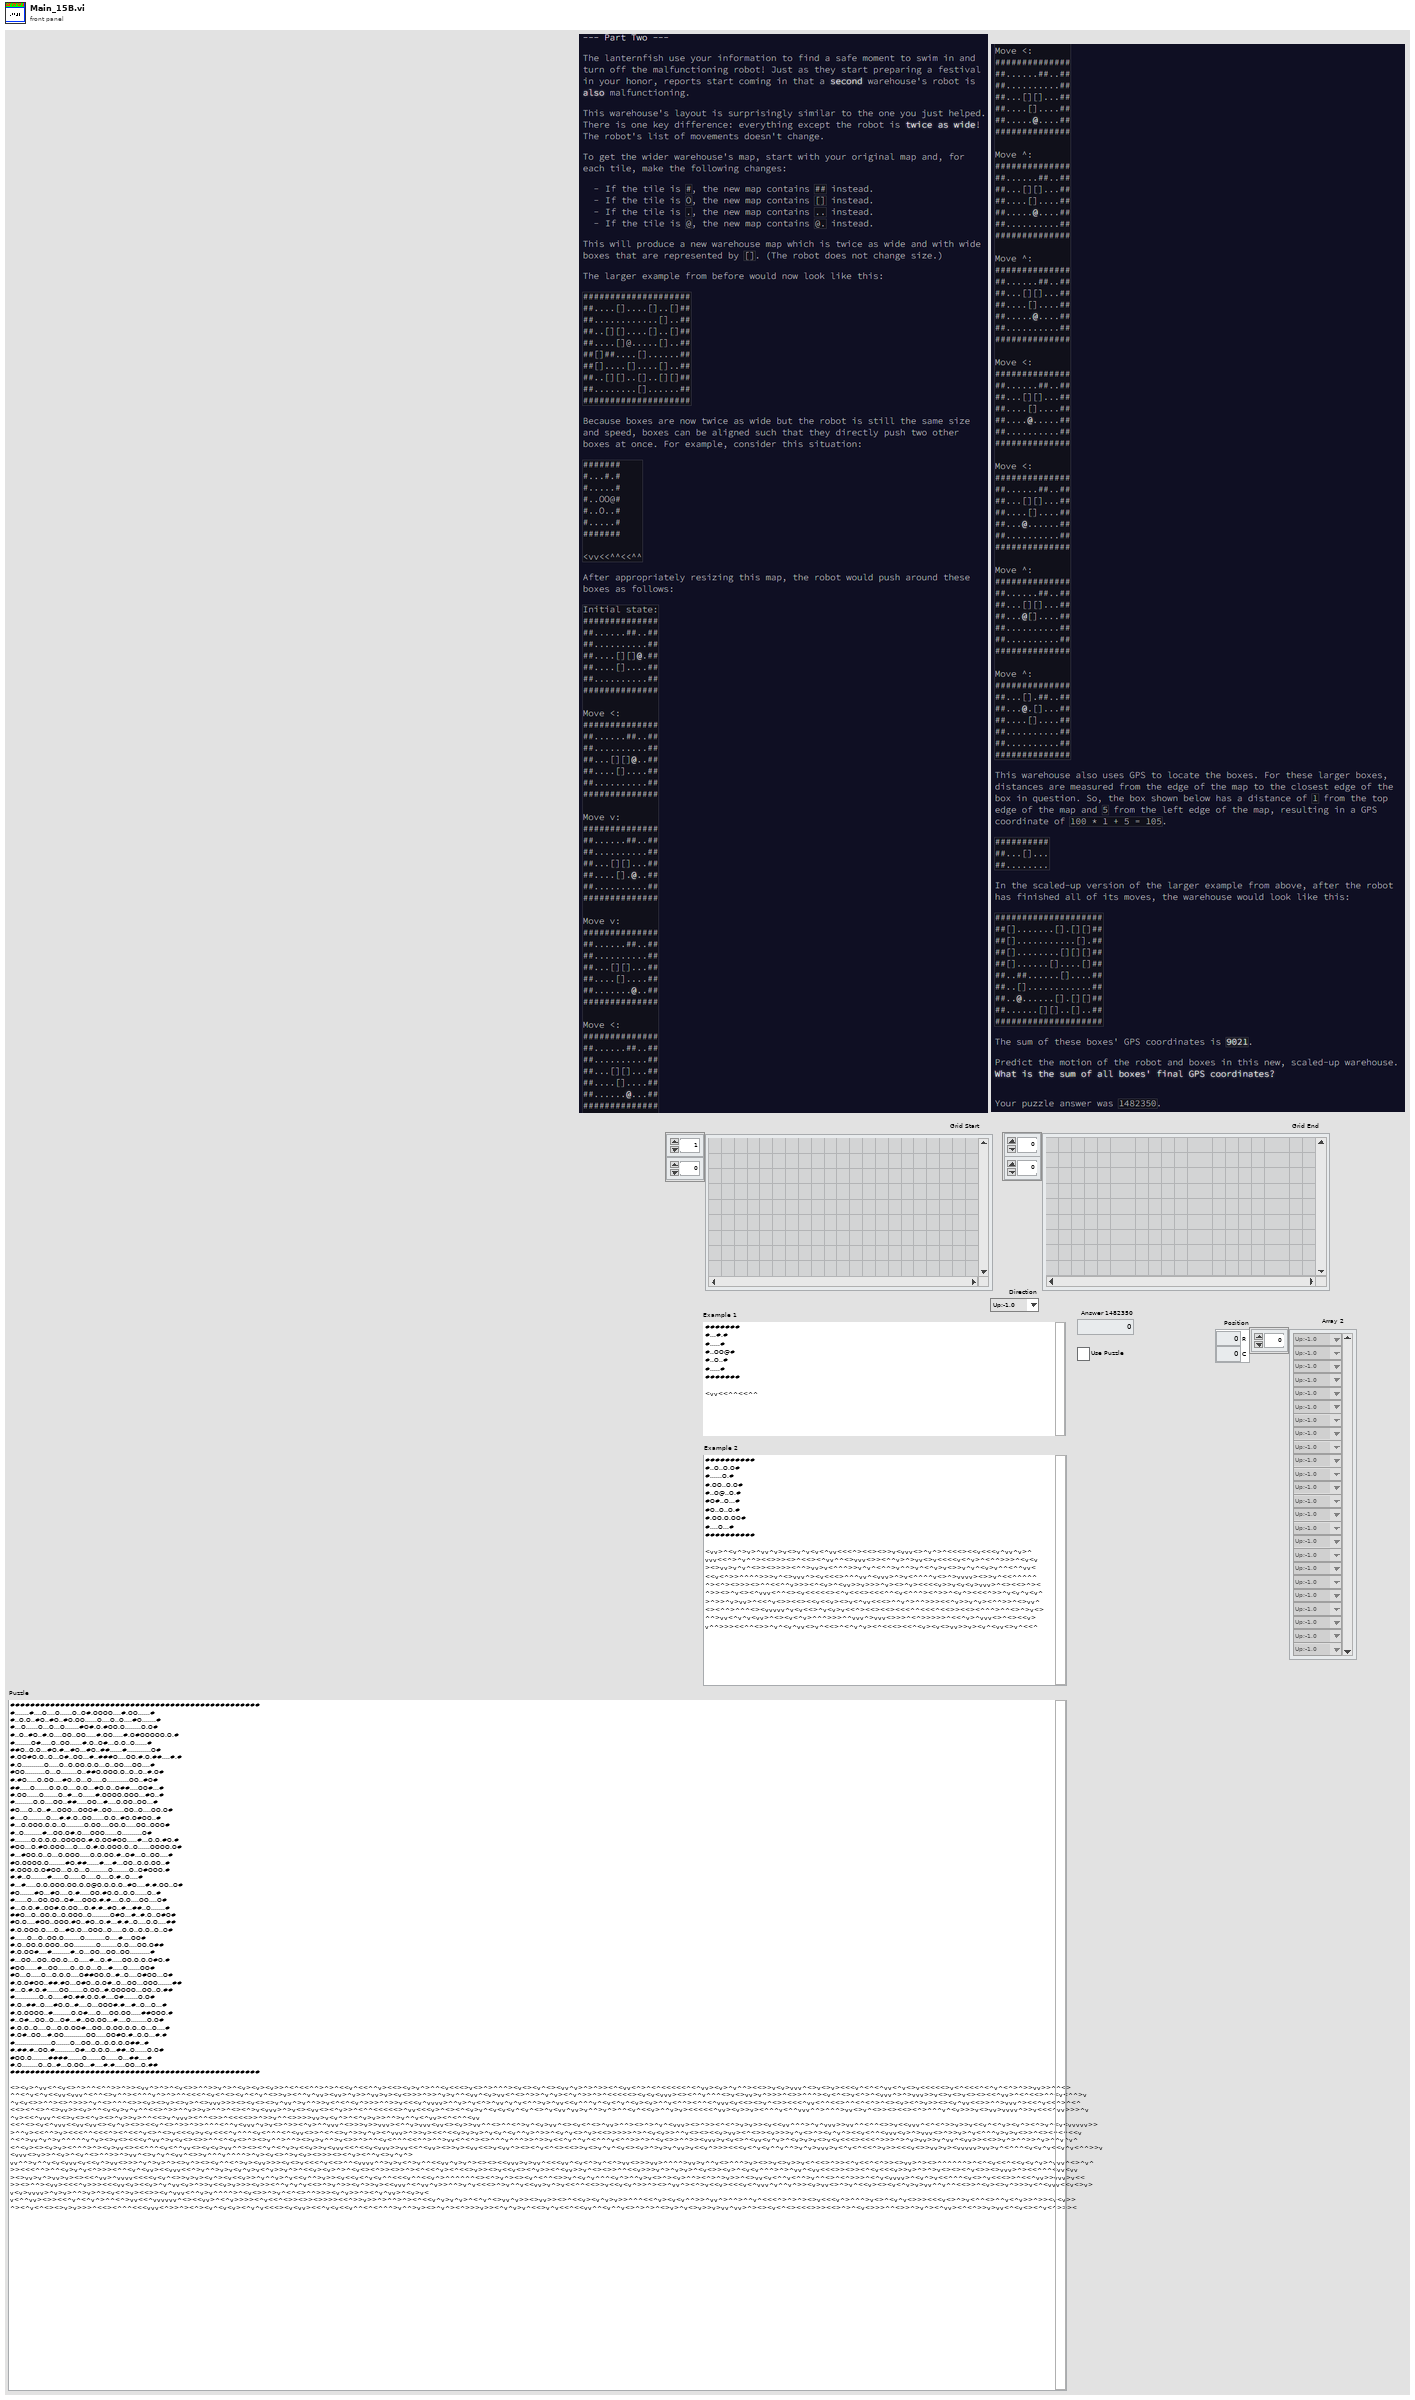
[diagram p1: front panel]
types:
  T1 = typedef "ENUM_4 Directions U-D-L-R.ctl" = enum16{"Up;-1,0", "Right;0,1", "Down;1,0", "Left;0,-1"}
  T2 = typedef "Cluster_Row-Column.ctl" = cluster{"R":i32, "C":i32}
  T3 = typedef "ENUM_Direction.ctl" = enum16{"Up;-1,0", "Right;0,1", "Down;1,0", "Left;0,-1"}
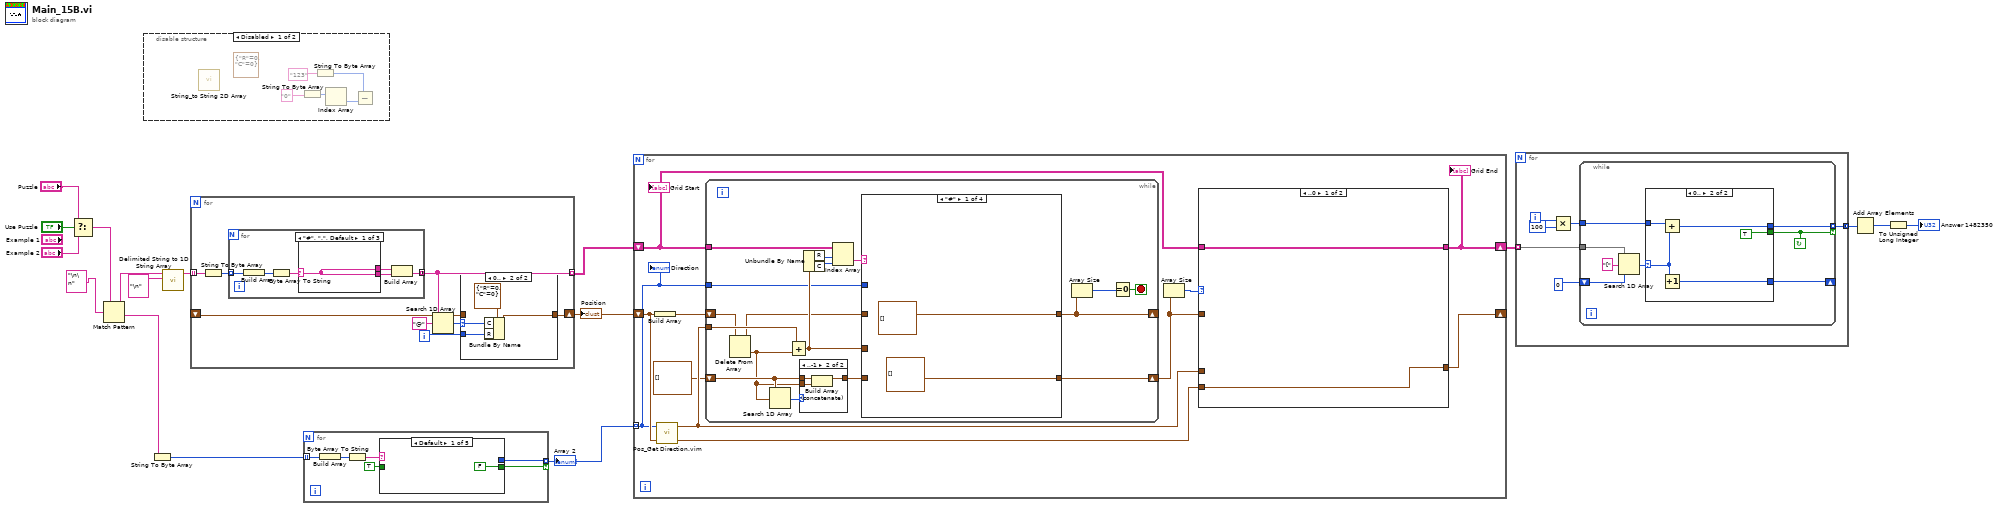
[diagram p0: block diagram]
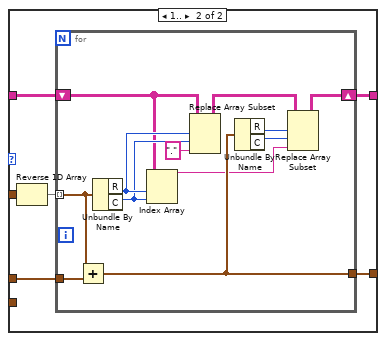
[diagram p3: hidden frame]
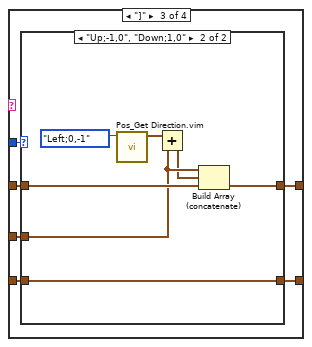
[diagram p6: hidden frame]
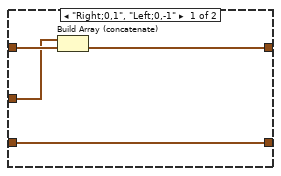
[diagram p7: hidden frame]
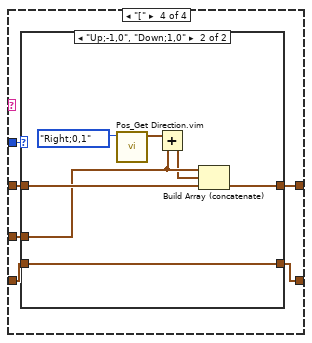
[diagram p8: hidden frame]
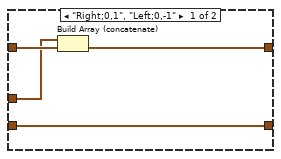
[diagram p9: hidden frame]
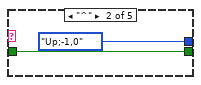
[diagram p10: hidden frame]
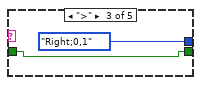
[diagram p11: hidden frame]
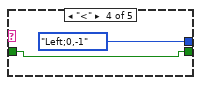
[diagram p12: hidden frame]
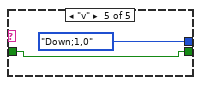
[diagram p13: hidden frame]
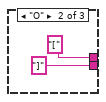
[diagram p16: hidden frame]
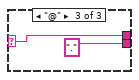
[diagram p17: hidden frame]
diagram:
  n1 = Select(t="Puzzle", s="Use Puzzle", f="Example 2") -> (s? t:f=w12:string)
  n2 = Match Pattern(string=w12, regular expression="\n\n" ("delimiter (Tab)")) -> (before substring=w11:string, after substring=w8:string)  [unwired: 1 in, 2 out]
  n3 = disable-structure shown="Disabled" {
    frame Disabled {
      (unwired) T2 {"R"=0, "C"=0} ("Position")
      n4 = call "String_to String 2D Array.vi"() -> ()  [unwired: 11 in, 1 out]
      n5 = String To Byte Array(string="0") -> (unsigned byte array=w20:u8[])
      n6 = String To Byte Array(string="123") -> (unsigned byte array=w18:u8[])
      n7 = Index Array(array=w20) -> (element=w19:u8)  [unwired: 1 in]
      n8 = Subtract(x=w18, y=w19) -> ()  [unwired: 1 out]
    }
    frame Enabled {
    }
  }
  n9 = String To Byte Array(string=w8) -> (unsigned byte array=w9:u8[])
  n10 = call <vilib>:"Delimited String to 1D String Array.vi"("delimiter"="\n" ("delimiter (Tab)"), "delimited string"=w11) -> ("string array"=w17:string[])  [unwired: 9 in]
  n11 = for {
    tunnel: w17 -> [w29] mode=indexing
    shift-right: [w25] -> w6
    shift-left: _ -> [w24]
    tunnel: [w23] -> w2 mode=indexing
    i -> [w26]
    n12 = String To Byte Array(string=w29) -> (unsigned byte array=w30:u8[])
    n13 = for {
      tunnel: w30 -> [w41] mode=indexing
      tunnel: [w36] -> w23 mode=concatenating
      n14 = Build Array(w41) -> (w40:u8[])
      n15 = Byte Array To String(unsigned byte array=w40) -> (string=w39:string)
      n16 = case shown="\"#\", \".\", Default" w39 {
        selector: w39 -> [w42 _ w45]
        tunnel: [w42 "[" w45] -> w38
        tunnel: [w42 "]" "."] -> w37
        frame "#", ".", Default {
        }
        frame "O" {
        }
        frame "@" {
        }
      }
      n17 = Build Array(w38, w37) -> (w36:string[])
    }
    n18 = Search 1D Array(1D array=w23, element="@") -> (index of element=w27:i32)  [unwired: 1 in]
    n19 = case shown="0.." w27 {
      selector: w27 -> [_ w34]
      tunnel: w26 -> [_ w33]
      tunnel: [w31 w32] -> w25
      tunnel: w24 -> [w31 _]
      frame ..-1 {
      }
      frame 0.. {
        n20 = Bundle By Name(cluster=T2 {"R"=0, "C"=0} ("Position"), "C"=w34, "R"=w33) -> (w32:T2)
      }
    }
  }
  "Position" <- w6
  n21 = for {
    tunnel: w9 -> [w52] mode=indexing
    tunnel: [w49] -> w7 mode=indexing if=w47
    n22 = Build Array(w52) -> (w51:u8[])
    n23 = Byte Array To String(unsigned byte array=w51) -> (string=w50:string)
    n24 = case shown="Default" w50 {
      tunnel: [_ ENUM_4_Directions_U-D-L-R."Up;-1,0" ("Direction") ENUM_4_Directions_U-D-L-R."Right;0,1" ("Direction") ENUM_4_Directions_U-D-L-R."Left;0,-1" ("Direction") ENUM_4_Directions_U-D-L-R."Down;1,0" ("Direction")] -> w49
      tunnel: [FALSE w54 w56 w58 w60] -> w47
      tunnel: TRUE -> [_ w54 w56 w58 w60]
      frame Default {
      }
      frame "^" {
      }
      frame ">" {
      }
      frame "<" {
      }
      frame "v" {
      }
    }
  }
  "Array 2" <- w7
  n25 = for {
    tunnel: w7 -> [w66] mode=indexing
    shift-right: [w63] -> w3
    shift-left: w2 -> [w62]
    shift-right: [w69] -> _
    shift-left: w6 -> [w67]
    n26 = Build Array(w67) -> (w71:T2[])
    n27 = call "Pos_Get Direction.vim"("Direction"=w66) -> ("Position"=w70:T2)  [unwired: 10 in]
    n28 = while {
      tunnel: w70 -> [w108]
      shift-right: [w98] -> _
      shift-left: w71 -> [w101]
      tunnel: w62 -> [w107]
      tunnel: w66 -> [w102]
      shift-right: [w99] -> w65
      shift-left: T2[] [] ("appended array") -> [w94]
      stop <- w96 stop-if-true
      n29 = Delete From Array(array=w101) -> (deleted portion=w92:T2, array with subset deleted=w100:T2[])  [unwired: 2 in]
      n30 = Search 1D Array(1D array=w94, element=w92) -> (index of element=w93:i32)  [unwired: 1 in]
      n31 = Add(x=w108, y=w92) -> (x+y=w103:T2)
      n32 = case shown="..-1" w93 {
        tunnel: [w109 w112] -> w95
        tunnel: w92 -> [_ w111]
        tunnel: w94 -> [w109 w110]
        frame 0.. {
        }
        frame ..-1 {
          n33 = Build Array (concatenate)(w110, w111) -> (w112:T2[])
        }
      }
      n34 = Unbundle By Name(w103) -> ("R"=w106:i32, "C"=w105:i32)
      n35 = Index Array(array=w107, index (row)=w106, index (col)=w105) -> (element=w104:string)
      n36 = case shown="\"#\"" w104 {
        tunnel: w100 -> [_ w116 w121 w138]
        tunnel: [T2[] [] w116 w119 w136] -> w98
        tunnel: w103 -> [_ _ w120 w137]
        tunnel: w102 -> [_ _ w122 w139]
        tunnel: [T2[] [] ("appended array") w115 w117 w134] -> w99
        tunnel: w95 -> [_ w115 w118 w135]
        frame "#" {
        }
        frame ".", Default {
        }
        frame "]" {
          n37 = case shown="\"Up;-1,0\", \"Down;1,0\"" w122 {
            tunnel: w121 -> [w126 w133]
            tunnel: w120 -> [w124 w128]
            tunnel: [w125 w132] -> w119
            tunnel: w118 -> [w123 w131]
            tunnel: [w123 w131] -> w117
            frame "Right;0,1", "Left;0,-1" {
              n38 = Build Array (concatenate)(w124, w126) -> (w125:T2[])
            }
            frame "Up;-1,0", "Down;1,0" {
              n39 = call "Pos_Get Direction.vim"("Direction"=ENUM_Direction."Left;0,-1") -> ("Position"=w129:T2)  [unwired: 10 in]
              n40 = Add(x=w129, y=w128) -> (x+y=w127:T2)
              n41 = Build Array (concatenate)(w128, w127, w133) -> (w132:T2[])
            }
          }
        }
        frame "[" {
          n42 = case shown="\"Up;-1,0\", \"Down;1,0\"" w139 {
            tunnel: w138 -> [w143 w150]
            tunnel: w137 -> [w141 w145]
            tunnel: [w142 w149] -> w136
            tunnel: w135 -> [w140 w148]
            tunnel: [w140 w148] -> w134
            frame "Right;0,1", "Left;0,-1" {
              n43 = Build Array (concatenate)(w141, w143) -> (w142:T2[])
            }
            frame "Up;-1,0", "Down;1,0" {
              n44 = call "Pos_Get Direction.vim"("Direction"=ENUM_Direction."Right;0,1") -> ("Position"=w146:T2)  [unwired: 10 in]
              n45 = Add(x=w146, y=w145) -> (x+y=w144:T2)
              n46 = Build Array (concatenate)(w145, w144, w150) -> (w149:T2[])
            }
          }
        }
      }
      n47 = Array Size(array=w98) -> (size(s)=w97:i32)
      n48 = Equal To 0?(x=w97) -> (x = 0?=w96:bool)
    }
    n49 = Array Size(array=w65) -> (size(s)=w68:i32)
    n50 = case shown="..0" w68 {
      tunnel: w65 -> [_ w79]
      tunnel: w62 -> [w73 w78]
      tunnel: [w73 w77] -> w63
      tunnel: w70 -> [_ w75]
      tunnel: [w72 w74] -> w69
      tunnel: w67 -> [w72 _]
      frame ..0 {
      }
      frame 1.. {
        n51 = Reverse 1D Array(array=w79) -> (reversed array=w76:T2[])
        n52 = for {
          tunnel: w76 -> [w87] mode=indexing
          shift-right: [w86] -> w77
          shift-left: w78 -> [w81]
          tunnel: w75 -> [w88]
          tunnel: [w85] -> w74
          n53 = Add(x=w87, y=w88) -> (x+y=w85:T2)
          n54 = Unbundle By Name(w87) -> ("R"=w91:i32, "C"=w90:i32)
          n55 = Index Array(array=w81, index (row)=w91, index (col)=w90) -> (element=w82:string)
          n56 = Replace Array Subset(array=w81, new element="." ("new element/subarray"), index (row)=w91, index (col)=w90) -> (w80:string[][])
          n57 = Unbundle By Name(w85) -> ("R"=w84:i32, "C"=w83:i32)
          n58 = Replace Array Subset(array=w80, new element=w82, index (row)=w84, index (col)=w83) -> (w86:string[][])
        }
      }
    }
    "Grid End" <- w63
    "Grid Start" <- w62
    "Direction" <- w66
  }
  n59 = for {
    tunnel: w3 -> [w154] mode=indexing
    tunnel: [w151] -> w5 mode=concatenating
    i -> [w156]
    n60 = Multiply(x=w156, y=100) -> (x*y=w152:i32)
    n61 = while {
      tunnel: w154 -> [w164]
      shift-right: [w157] -> _
      shift-left: 0 -> [w161]
      tunnel: w152 -> [w160]
      tunnel: [w159] -> w151 mode=indexing if=w158
      stop <- w158 continue-if-true
      n62 = Search 1D Array(1D array=w164, element="[", start index (0)=w161) -> (index of element=w162:i32)
      n63 = case shown="0.." w162 {
        selector: w162 -> [_ w165]
        tunnel: w160 -> [_ w169]
        tunnel: [_ w168] -> w159
        tunnel: [_ TRUE] -> w158
        tunnel: [_ w166] -> w157
        frame ..-1 {
        }
        frame 0.. {
          n64 = Add(x=w169, y=w165) -> (x+y=w168:i32)
          n65 = Increment(x=w165) -> (x+1=w166:i32)
        }
      }
    }
  }
  n66 = Add Array Elements(numeric array=w5) -> (sum=w4:i32)
  n67 = To Unsigned Long Integer(number=w4) -> (unsigned 32bit integer=→"Answer 1482350":u32)
